vi "Motor.vi"(8 "error in Linx":errorcluster, 9 "LINX Ref":T1, 10 "Motor_Right":dbl, 11 "Motor_Left":dbl) -> (0 "error out":errorcluster, 3 "LINX Resource":T1)   [LabVIEW 2013]
uses:
  <vilib>/LabVIEW Hacker/LINX/Private/Type Defs/LINX Ref.ctl
  <vilib>/LabVIEW Hacker/LINX/Private/Type Defs/Platform.ctl
  <vilib>/LabVIEW Hacker/LINX/Private/Type Defs/Interface.ctl
  <vilib>/LabVIEW Hacker/LINX/Private/Device/Type Defs/LINX Device Config.ctl
  <vilib>/LabVIEW Hacker/LINX/Private/Device/Type Defs/TCP Config.ctl
  <vilib>/LabVIEW Hacker/LINX/Private/Type Defs/Device Family.ctl
  <vilib>/LabVIEW Hacker/LINX/Public/Peripherals/PWM/Set Duty Cycle 1 Chan.vi
  <vilib>/LabVIEW Hacker/LINX/LVH-LINX.lvlib
  <vilib>/LabVIEW Hacker/LINX/Private/Device/Device.lvlib
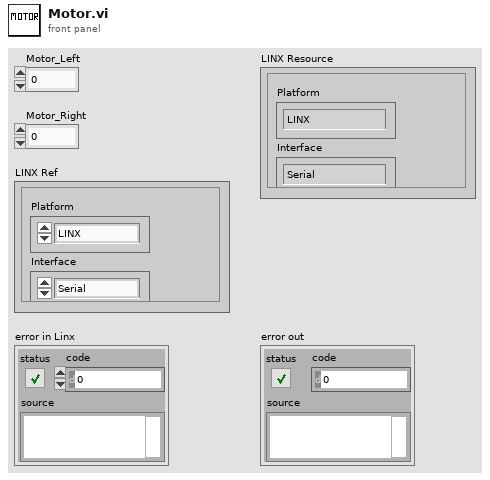
[diagram p1: front panel]
types:
  T1 = typedef "LVH-LINX.lvlib/LINX Ref.ctl" = cluster{"Platform":T2, "Interface":T3, "LINX Device Config":T4}
  T2 = typedef "LVH-LINX.lvlib/Platform.ctl" = enum16{"LINX", "myRIO"}
  T3 = typedef "LVH-LINX.lvlib/Interface.ctl" = enum16{"Serial", "TCP"}
  T4 = typedef "LVH-LINX.lvlib/Device.lvlib/LINX Device Config.ctl" = cluster{"Interface":T3, "COM Port":refnum<visa-resource-name>, "TCP Configuration":T5, "Device Family":T6, "Device ID":u8, "Device Name":string, "TCP Ref":refnum<k5>}
  T5 = typedef "LVH-LINX.lvlib/Device.lvlib/TCP Config.ctl" = cluster{"IP Address":string, "Port":u16}
  T6 = typedef "LVH-LINX.lvlib/Device Family.ctl" = enum8{"National Instruments", "Digilent", "Arduino"}
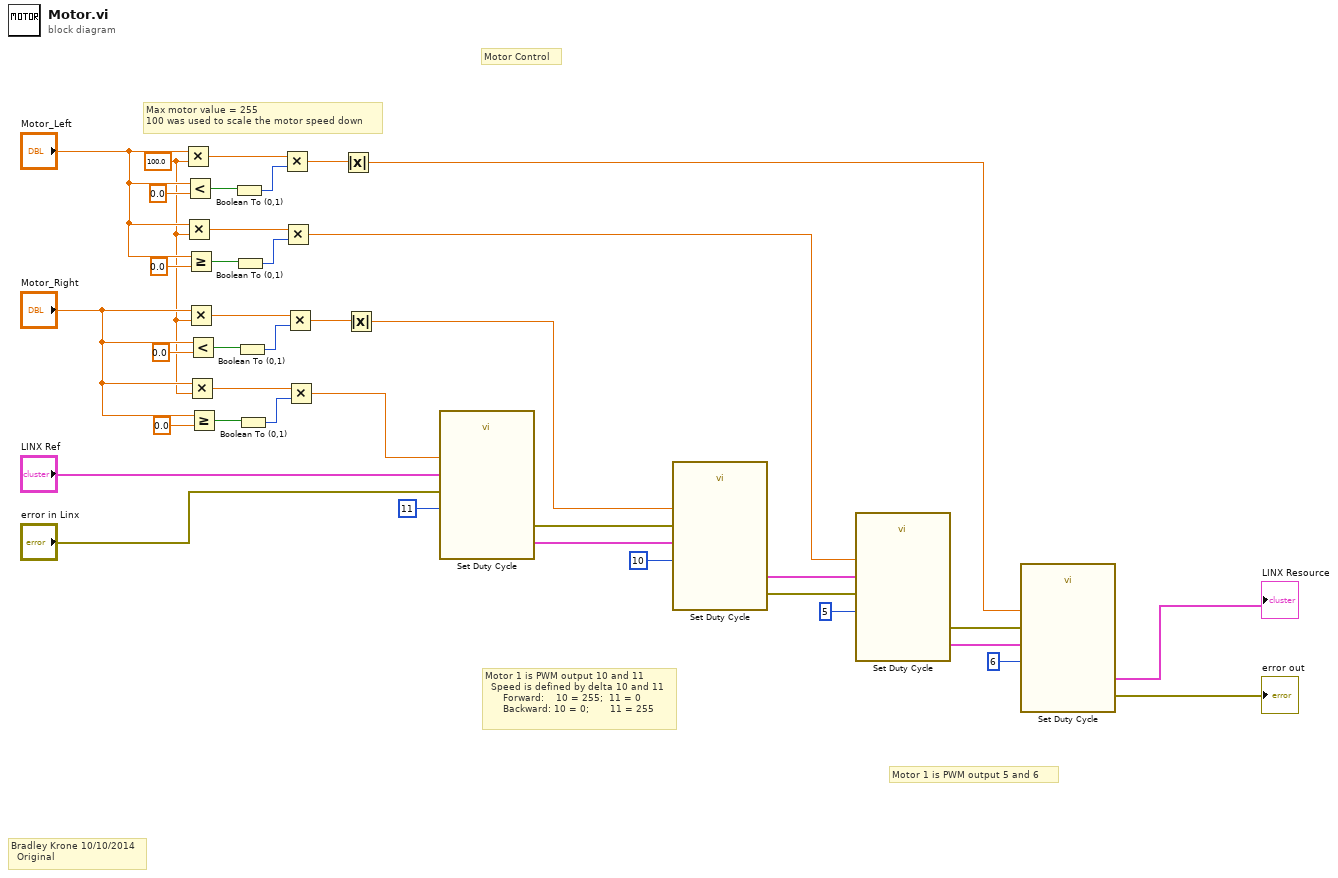
[diagram p0: block diagram]
diagram:
  w1 = 100.0 ("y")
  # "Motor 1 is PWM output 5 and 6"
  # "Motor 1 is PWM output 10 and 11\n  Speed is defined by delta 10 and 11\n      Forward:    10 = 255;  11 = 0\n      Backward: 10 = 0;       11 = 255"
  # "Max motor value = 255\n100 was used to scale the motor speed down"
  # "Bradley Krone 10/10/2014\n  Original"
  # "Motor Control"
  n1 = Multiply(x="Motor_Left", y=w1) -> (x*y=w31:dbl)
  n2 = Multiply(x="Motor_Left", y=w1) -> (x*y=w28:dbl)
  n3 = Less?(x="Motor_Left", y=0.0) -> (x < y?=w32:bool)
  n4 = Greater Or Equal?(x="Motor_Left", y=0.0) -> (x >= y?=w27:bool)
  n5 = Multiply(x="Motor_Right", y=w1) -> (x*y=w14:dbl)
  n6 = Multiply(x="Motor_Right", y=w1) -> (x*y=w10:dbl)
  n7 = Less?(x="Motor_Right", y=0.0) -> (x < y?=w15:bool)
  n8 = Greater Or Equal?(x="Motor_Right", y=0.0) -> (x >= y?=w9:bool)
  n9 = Boolean To (0,1)(Boolean=w32) -> (0, 1=w30:i16)
  n10 = Boolean To (0,1)(Boolean=w27) -> (0, 1=w29:i16)
  n11 = Boolean To (0,1)(Boolean=w15) -> (0, 1=w13:i16)
  n12 = Boolean To (0,1)(Boolean=w9) -> (0, 1=w11:i16)
  n13 = Multiply(x=w31, y=w30) -> (x*y=w34:dbl)
  n14 = Multiply(x=w28, y=w29) -> (x*y=w36:dbl)
  n15 = Multiply(x=w14, y=w13) -> (x*y=w17:dbl)
  n16 = Multiply(x=w10, y=w11) -> (x*y=w12:dbl)
  n17 = Absolute Value(x=w34) -> (abs(x)=w37:dbl)
  n18 = Absolute Value(x=w17) -> (abs(x)=w18:dbl)
  n19 = call-poly <vilib>:"Set Duty Cycle.vi"("Error In"="error in Linx", "Duty Cycle"=w12, "PWM Channel"=u8 11 ("Digital Output Channel"), "LINX Resource"="LINX Ref") -> ("Error Out"=w4:errorcluster, "LINX Resource"=w5:T1)  [unwired: 6 in]
  n20 = call-poly <vilib>:"Set Duty Cycle.vi"("Error In"=w4, "Duty Cycle"=w18, "PWM Channel"=u8 10 ("Digital Output Channel 2"), "LINX Resource"=w5) -> ("Error Out"=w21:errorcluster, "LINX Resource"=w20:T1)  [unwired: 6 in]
  n21 = call-poly <vilib>:"Set Duty Cycle.vi"("Error In"=w21, "Duty Cycle"=w36, "PWM Channel"=u8 5 ("Digital Output Channel"), "LINX Resource"=w20) -> ("Error Out"=w22:errorcluster, "LINX Resource"=w23:T1)  [unwired: 6 in]
  n22 = call-poly <vilib>:"Set Duty Cycle.vi"("Error In"=w22, "Duty Cycle"=w37, "PWM Channel"=u8 6 ("Digital Output Channel"), "LINX Resource"=w23) -> ("Error Out"=→"error out":errorcluster, "LINX Resource"=→"LINX Resource":T1)  [unwired: 6 in]
